vi "etlUSBWrite.vi"(1 "mode":u16(ring) items=["position (um)", "1/focal length (dpt)"], 2 "lens":enum16{"0", "1"}(ring), 3 "input":dbl) -> ()   [LabVIEW 2017]
uses:
  globalDevices.vi
panel:
  out "concatenated string":string
  out "return count":u32
  out "read buffer":string
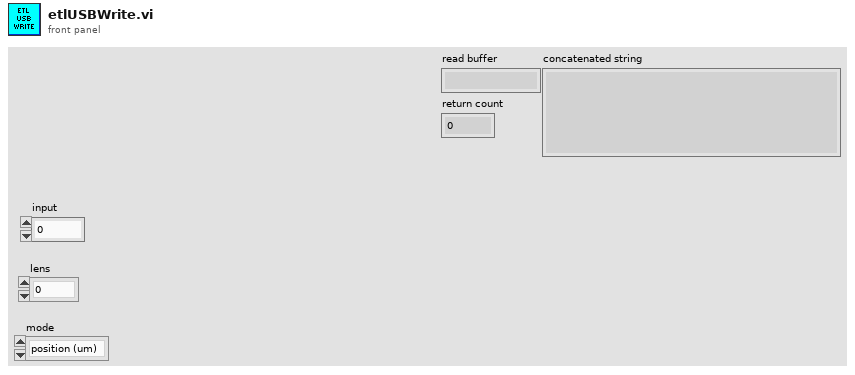
[diagram p1: front panel]
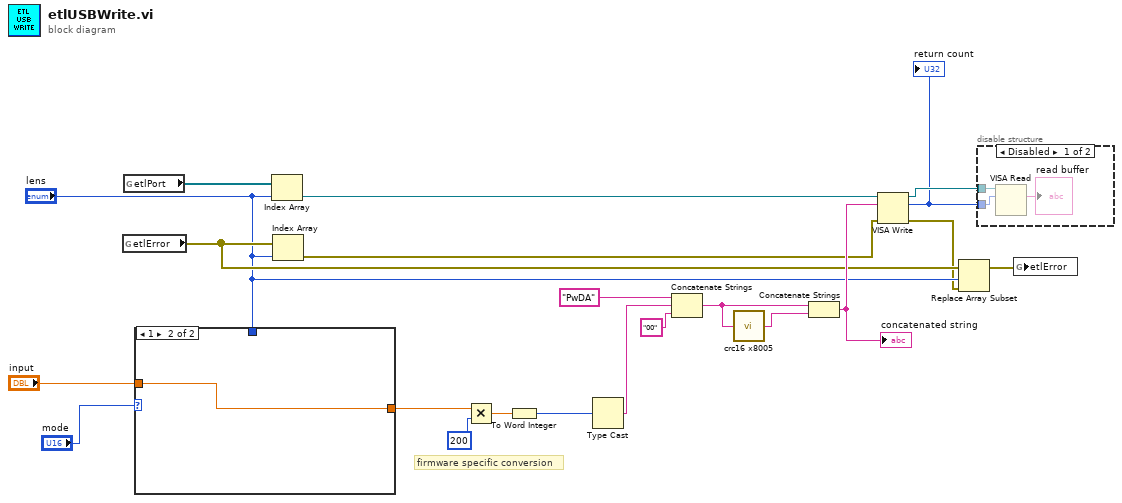
[diagram p0: block diagram]
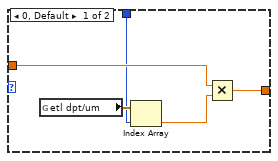
[diagram p3: hidden frame]
diagram:
  # "firmware specific conversion"
  n1 = global read "globalDevices.vi" "etlError"() -> (w8:errorcluster[])
  n2 = global read "globalDevices.vi" "etlPort"() -> (w21:refnum<visa-resource-name>[])
  n3 = case shown="1" "mode" {
    tunnel: "input" -> [w26 w27]
    tunnel: [w23 w27] -> w1
    tunnel: "lens" -> [w22 _]
    frame 0, Default {
      n4 = global read "globalDevices.vi" "etl dpt/um"() -> (w25:dbl[])
      n5 = Index Array(array=w25, index=w22) -> (element=w24:dbl)
      n6 = Multiply(x=w26, y=w24) -> (x*y=w23:dbl)
    }
    frame 1 {
    }
  }
  n7 = Index Array(array=w21, index="lens") -> (element=w20:refnum<visa-resource-name>)
  n8 = Index Array(array=w8, index="lens") -> (element=w9:errorcluster)
  n9 = Multiply(x=w1, y=u16 200) -> (x*y=w17:dbl)
  n10 = To Word Integer(number=w17) -> (16bit integer=w16:i16)
  n11 = Type Cast(x=w16) -> (*(type *) &x=w14:string)  [unwired: 1 in]
  n12 = Concatenate Strings("PwDA", w14, "00" ("string")) -> (w12:string)
  n13 = call "crc16 x8005.vi"("message"=w12) -> ("CRC16"=w11:string)  [unwired: 4 in]
  n14 = Concatenate Strings(w12, w11) -> (w10:string)
  "concatenated string" <- w10
  n15 = VISA Write(VISA resource name=w20, write buffer=w10, error in (no error)=w9) -> (VISA resource name out=w3:refnum<visa-resource-name>, return count=w2:u32, error out=w6:errorcluster)
  "return count" <- w2
  n16 = Replace Array Subset(array=w8, new element=w6, index="lens") -> (w4:errorcluster[])
  n17 = disable-structure shown="Disabled" {
    disable-tunnel: w3 -> [w30 _]
    disable-tunnel: w2 -> [w29 _]
    frame Disabled {
      n18 = VISA Read(VISA resource name=w30, byte count=w29) -> (read buffer=→"read buffer":string)  [unwired: 1 in, 3 out]
    }
    frame Enabled {
    }
  }
  n19 = global write "globalDevices.vi" "etlError"(w4) -> ()
